vi "Initialize Status Channels.vi"(8 "error in (no error)":errorcluster, 11 "VeriStand Data Sharing Framework in":refnum<class "VeriStand DSF.lvclass">) -> (0 "error out":errorcluster, 1 "status channels refs":T1[](array[typedef]) format="%.0x", 2 "status channel offsets":u64[](array[numeric]) format="%.0x", 3 "VeriStand Data Sharing Framework out":refnum<class "VeriStand DSF.lvclass">)   [LabVIEW 2017, in "DSF Engine.lvlib" / "VeriStand DSF.lvclass"]
uses:
  VeriStand DSF.lvclass
  <vilib>/NI Veristand/Custom Device API/Custom Device Item Ref.ctl
  VeriStand DSF.lvclass/VeriStand DSF.ctl
  <vilib>/NI Veristand/Custom Device API/Data Access Type.ctl
  <vilib>/NI Veristand/Custom Device API/Custom Device API.lvlib
  Shared/DSF Shared.lvlib
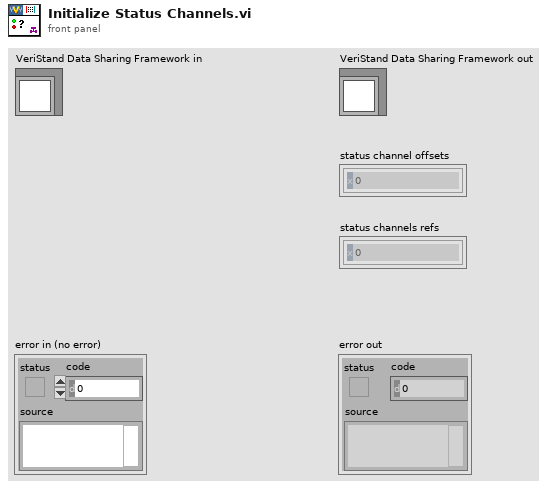
[diagram p1: front panel]
types:
  T1 = typedef "Custom Device API.lvlib/Custom Device Item Ref.ctl" = u64
  T2 = typedef "Custom Device API.lvlib/Data Access Type.ctl" = enum16{"Read", "Write"}
  T3 = typedef "Custom Device API.lvlib/Data Reference.ctl" = i32
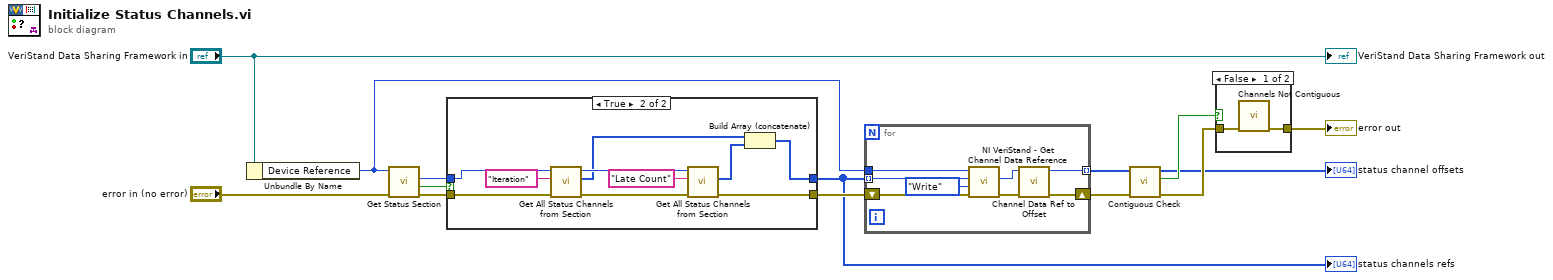
[diagram p0: block diagram]
diagram:
  n1 = Unbundle By Name("VeriStand Data Sharing Framework in") -> ("Device Reference"=w8:T1)
  n2 = call "Get Status Section.vi"("error in (no error)"="error in (no error)", "Item Ref in"=w8) -> ("error out"=w13:errorcluster, "found"=w4:bool, "Status Section ref"=w12:T1)  [unwired: 6 in, 1 out]
  n3 = case shown="True" w4 {
    tunnel: w13 -> [w15 w24]
    tunnel: w12 -> [_ w23]
    tunnel: [w15 w16] -> w11
    tunnel: [_ w25] -> w3
    frame False {
    }
    frame True {
      n4 = call "Get All Status Channels from Section.vi"("error in (no error)"=w24, "Section Name"="Iteration", "Item Ref in"=w23) -> ("error out"=w20:errorcluster, "status channels refs"=w18:T1[], "Item Ref out"=w21:T1)  [unwired: 6 in]
      n5 = call "Get All Status Channels from Section.vi"("error in (no error)"=w20, "Section Name"="Late Count", "Item Ref in"=w21) -> ("error out"=w16:errorcluster, "status channels refs"=w17:T1[])  [unwired: 6 in, 1 out]
      n6 = Build Array (concatenate)(w18, w17) -> (w25:T1[])
    }
  }
  "status channels refs" <- w3
  n7 = for {
    shift-right: [w32] -> w10
    shift-left: w11 -> [w31]
    tunnel: [w29] -> w9 mode=indexing
    tunnel: w8 -> [w27]
    tunnel: w3 -> [w26] mode=indexing
    n8 = call <vilib>:"NI VeriStand - Get Channel Data Reference.vi"("error in (no error)"=w31, "Access"=Data_Access_Type."Write", "Channel Ref in"=w26, "Device Ref in"=w27) -> ("error out"=w33:errorcluster, "Channel Data Reference"=w30:T3)  [unwired: 5 in, 1 out]
    n9 = call "Channel Data Ref to Offset.vi"("error in (no error)"=w33, "Channel Data Reference"=w30) -> ("error out"=w32:errorcluster, "channel offset"=w29:u64)  [unwired: 8 in]
  }
  n10 = call "Contiguous Check.vi"("error in (no error)"=w10, "channel offsets in"=w9) -> ("error out"=w6:errorcluster, "contiguous?"=w5:bool, "channel offsets out"=→"status channel offsets":u64[])  [unwired: 7 in]
  n11 = case shown="False" w5 {
    tunnel: [w35 w36] -> w7
    tunnel: w6 -> [w34 w36]
    frame False {
      n12 = call "Channels Not Contiguous.vi"("error in (no error)"=w34) -> ("error out"=w35:errorcluster)  [unwired: 10 in]
    }
    frame True {
    }
  }
  "error out" <- w7
  "VeriStand Data Sharing Framework out" <- "VeriStand Data Sharing Framework in"
